vi "replace cursor.vi"(7 "action":enum16{"", "read", "write"}(ring)=enum."write", 8 "cursor index":i32, 9 "new  Y":dbl=nan, 10 "new X":dbl=nan, 11 "Cursor List in":T1) -> (1 "read Y":dbl, 2 "read X":dbl, 3 "Cursor List Out":T1)   [LabVIEW 2021]
uses:
  <vilib>/Utility/miscctls.llb/LVCursorListTypeDef.ctl
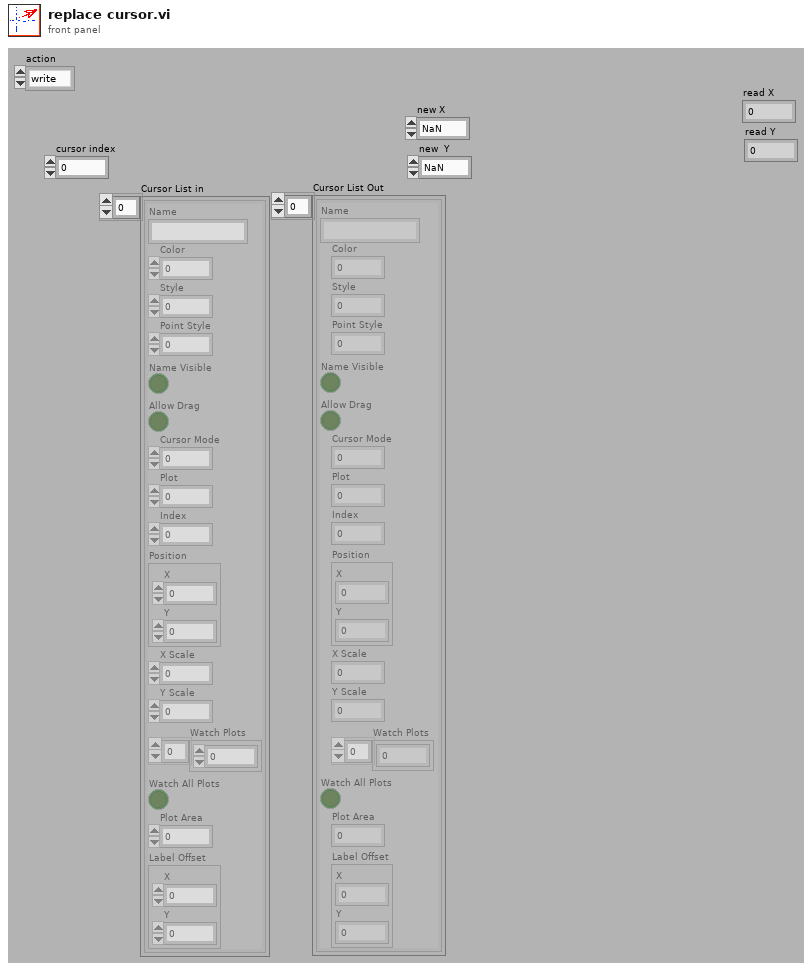
[diagram p1: front panel]
types:
  T1 = typedef "LVCursorListTypeDef.ctl" = cluster{"Name":string, "Color":u32, "Style":u8, "Point Style":u8, "Name Visible":bool, "Allow Drag":bool, "Cursor Mode":u32, "Plot":i32, "Index":i32, "Position":cluster{"X":dbl, "Y":dbl}, "X Scale":u32, "Y Scale":u32, "Watch Plots":i32[], "Watch All Plots":bool, "Plot Area":i32, "Label Offset":cluster{"X":dbl, "Y":dbl}}[]
  T2 = cluster{"Name":string, "Color":u32, "Style":u8, "Point Style":u8, "Name Visible":bool, "Allow Drag":bool, "Cursor Mode":u32, "Plot":i32, "Index":i32, "Position":cluster{"X":dbl, "Y":dbl}, "X Scale":u32, "Y Scale":u32, "Watch Plots":i32[], "Watch All Plots":bool, "Plot Area":i32, "Label Offset":cluster{"X":dbl, "Y":dbl}}
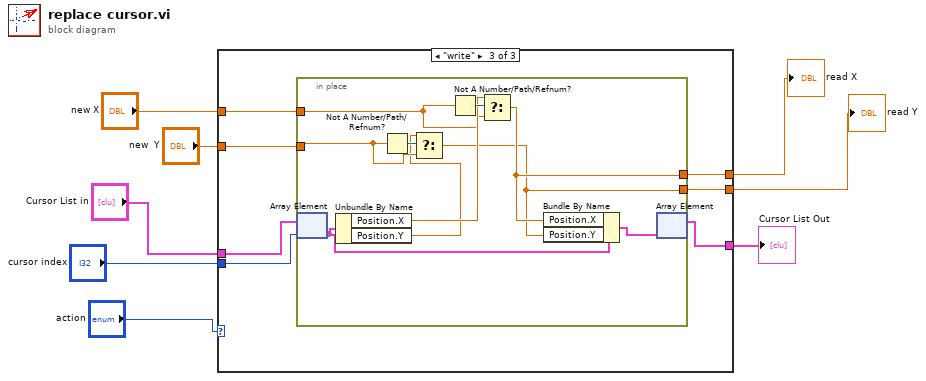
[diagram p0: block diagram]
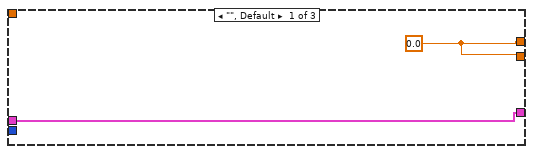
[diagram p2: hidden frame]
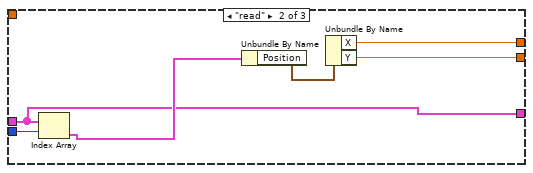
[diagram p3: hidden frame]
diagram:
  n1 = case shown="\"write\"" "action" {
    tunnel: "cursor index" -> [_ w15 w19]
    tunnel: "Cursor List in" -> [w10 w13 w21]
    tunnel: [w10 w13 w20] -> w6
    tunnel: "new  Y" -> [_ _ w22]
    tunnel: "new X" -> [_ _ w23]
    tunnel: [w9 w12 w18] -> w2
    tunnel: [w9 w11 w17] -> w1
    frame "", Default {
      w9 = 0.0
    }
    frame "read" {
      n2 = Index Array(array=w13, index=w15) -> (element=w16:T2)
      n3 = Unbundle By Name(w16) -> ("Position"=w14:cluster{"X":dbl, "Y":dbl})
      n4 = Unbundle By Name(w14) -> ("X"=w12:dbl, "Y"=w11:dbl)
    }
    frame "write" {
      n5 = in-place {
        in-place-border: w23 -> [w29]
        in-place-border: w22 -> [w27]
        in-place-border: [w25] -> w18
        in-place-border: [w24] -> w17
        n6 = in-place-array #1(w21, w19) -> (w33:T2)
        n7 = Unbundle By Name(w33) -> ("Position.X"=w30:dbl, "Position.Y"=w26:dbl)
        n8 = Not A Number/Path/Refnum?(number/path/refnum=w27) -> (NaN/Path/Refnum?=w28:bool)
        n9 = Select(t=w26, s=w28, f=w27) -> (s? t:f=w24:dbl)
        n10 = Not A Number/Path/Refnum?(number/path/refnum=w29) -> (NaN/Path/Refnum?=w31:bool)
        n11 = Select(t=w30, s=w31, f=w29) -> (s? t:f=w25:dbl)
        n12 = Bundle By Name(cluster=w33, "Position.X"=w25, "Position.Y"=w24) -> (w32:T2)
        n13 = in-place-array #1(w32) -> (w20:T1)  [unwired: 1 out]
      }
    }
  }
  "Cursor List Out" <- w6
  "read X" <- w2
  "read Y" <- w1
